vi "Test Case.Serialize - Invalid character in Classname - XML does not contain invalid character.vi"() -> ()   [LabVIEW 2013, in "JUnit XML Tests.lvlib"]
uses:
  JUnit XML Tests.lvlib
  <vilib>/xml/Close Reference(Node).vi
  <vilib>/addons/_JKI Toolkits/Caraya/classes/Assert/Assert Equal Value_Variant.vi
  JUnit XML/JUnit XML.lvlib
  <vilib>/addons/_JKI Toolkits/Caraya/classes/Test/Test.lvclass
  <vilib>/addons/_JKI Toolkits/Caraya/classes/Assert/Assert.lvclass
  <resource>/objmgr/DOMUserDefRef.rc
  <vilib>/xml/NI_XML.lvlib
  JUnit XML/Test Case/Test Case.lvclass
panel:
  out "error out":errorcluster
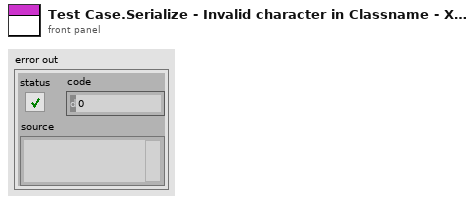
[diagram p1: front panel]
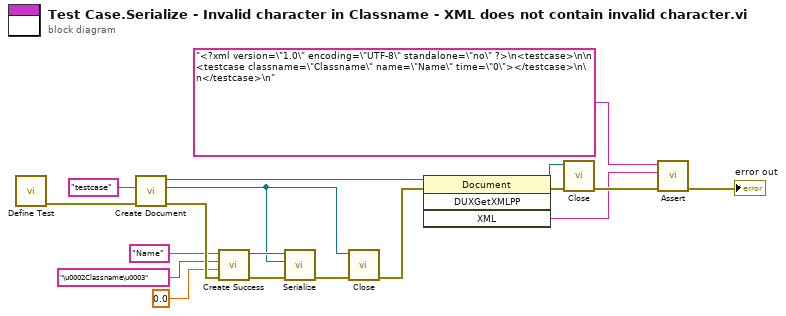
[diagram p0: block diagram]
diagram:
  n1 = call <vilib>:"Define Test.vi"() -> ("error out"=w18:errorcluster)  [unwired: 10 in, 1 out]
  n2 = call "Create Document.vi"("error in (no error)"=w18, "Root Element Name"="testcase") -> ("error out"=w14:errorcluster, "Root Element"=w10:refnum<k20>, "Document"=w13:refnum<k20>)  [unwired: 7 in]
  n3 = call "Create Success.vi"("error in (no error)"=w14, "Time"=0.0, "Classname"="\u0002Classname\u0003", "Name"="Name") -> ("error out"=w16:errorcluster, "Test Case"=w17:refnum<class "Test Case.lvclass">)  [unwired: 6 in]
  n4 = call "Serialize.vi"("error in (no error)"=w16, "Element in"=w10, "Test Case in"=w17) -> ("error out"=w12:errorcluster)  [unwired: 7 in, 1 out]
  n5 = call-poly <vilib>:"Close.vi"("error in (no error)"=w12, "node"=w10) -> ("error out"=w11:errorcluster)  [unwired: 7 in]
  n6 = invoke class="Document" method="DUXGetXMLPP"(reference=w13, error in=w11) -> (reference out=w8:refnum<k20>, error out=w9:errorcluster, "XML"=w6:string)  [unwired: 2 in, 1 out]
  n7 = call-poly <vilib>:"Close.vi"("error in (no error)"=w9, "node"=w8) -> ("error out"=w7:errorcluster)  [unwired: 7 in]
  n8 = call-poly <vilib>:"Assert.vi"("error in (no error)"=w7, "Actual"=w6, "Expected"="<?xml version=\"1.0\" encoding=\"UTF-8\" standalone=\"no\" ?>\n<testcase>\n\n  <testcase classname=\"Classname\" name=\"Name\" time=\"0\"></testcase>\n\n</testcase>\n") -> ("error out"=→"error out":errorcluster)  [unwired: 7 in, 1 out]
